vi "4-5.vi"(1 "数值":dbl) -> (0 "数值 2":i32)   [LabVIEW 2017]
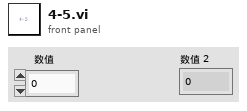
[diagram p1: front panel]
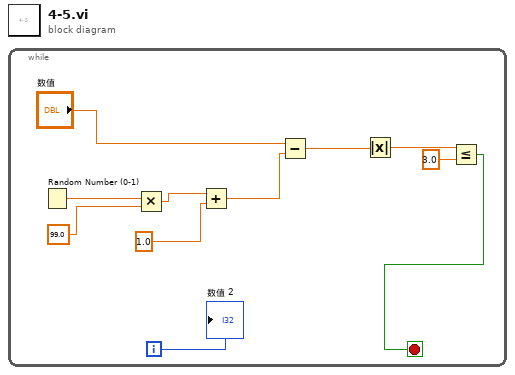
[diagram p0: block diagram]
diagram:
  n1 = while {
    i -> [w11]
    stop <- w1 stop-if-true
    n2 = Random Number (0-1)() -> (number: 0 to 1=w5:dbl)
    n3 = Multiply(x=w5, y=99.0) -> (x*y=w6:dbl)
    n4 = Add(x=w6, y=1.0) -> (x+y=w8:dbl)
    n5 = Subtract(x="数值", y=w8) -> (x-y=w9:dbl)
    n6 = Absolute Value(x=w9) -> (abs(x)=w10:dbl)
    n7 = Less Or Equal?(x=w10, y=3.0) -> (x <= y?=w1:bool)
    "数值 2" <- w11
  }
